vi "CSM - Module VI Reference.vi"(6 "Response Timeout (-2 Using Global Settings)":i32=-2, 7 "Current Module (\"\" to Generate an ID)":string, 8 "error in (no error)":errorcluster, 9 "Force? (F)":bool, 11 "CSM Name":string) -> (0 "error out":errorcluster, 3 "CSM Module VIRef":refnum<vi>)   [LabVIEW 2017, in "Communicable State Machine.lvlib"]
doc: "Obtains the VI Reference of the input module.\n\nThe following is the logic of this VI:\n- This VI queries and retrieves the CSM module's VI reference by sending a `VI Reference` synchronous message, so it has input parameters similar to the VI that sends synchronous messages.\n- This VI caches the VI reference of the CSM module queried during the current main program run in the background. When the same module is queried again and the retrieved VI reference is still valid, the cached VI reference is returned directly instead of sending another synchronous message query.\n- If you need to force a re-query of the module's VI reference, you can set <b>Force? (F)</b> to TRUE.\n\nBehavior for CSM in special operation modes:\n- <b>Worker Mode</b>: Returns the VI reference of the worker node handling the `VI Reference` message.\n- <b>Chain of Responsibility Mode</b>: Returns the VI reference of the first node of the CSM module in Chain of Responsibility Mode.\n- <b>System-Level Module</b>: Same as normal mode CSM. Returns the VI reference of the system-level module.\n\n\n> [!WARNING] <b>Multiple CSMs in a Single VI</b>\n>\n> - It is not recommended to place multiple (>=2) CSMs in a flat layout within a single VI. While this will not cause logical issues in the program, it will prevent the CSM Debug Console from loading all the inner and outer interfaces of the flat CSMs in that VI - only one will be loaded.\n\n\n-- <b>Controls</b> --\n- <b>Current Module (\"\" to Generate an ID)</b>: Tag for the querying CSM module. If empty, a unique ID is generated.\n- <b>CSM Name</b>: CSM module name.\n- <b>Force? (F)</b>: Whether to force a re-query of the module's VI reference. The default is FALSE.\n- <b>Response Timeout (-2 Using Global Settings)</b>: Timeout for synchronous calls. The default is -2, which uses the global setting. You can set the global timeout using the CSM - Set TMO of Sync-Reply VI.\n\n-- <b>Indicators</b> --\n- <b>CSM Module VIRef</b>: VI reference of the CSM module."
uses:
  Communicable State Machine.lvlib
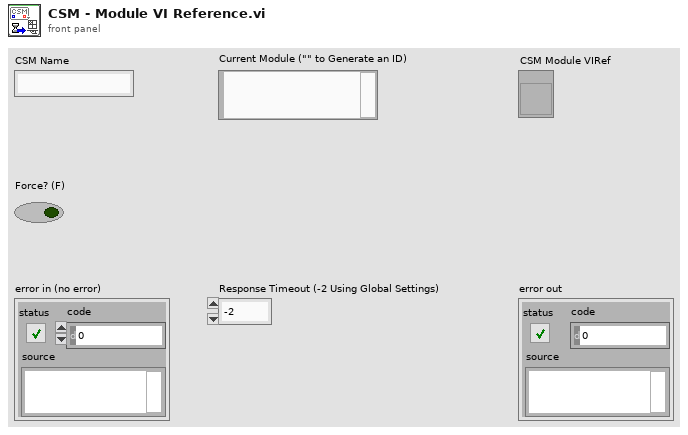
[diagram p1: front panel]
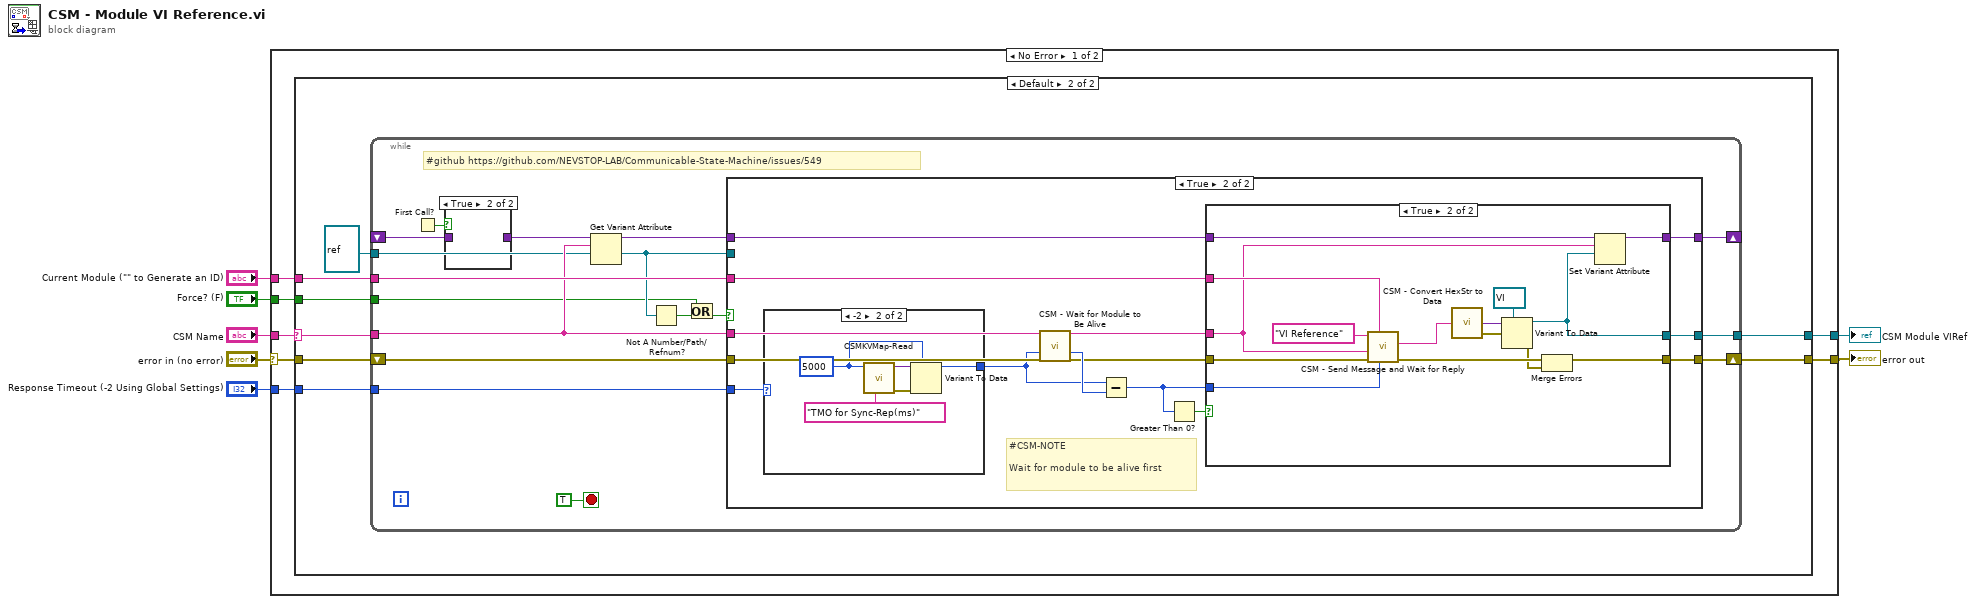
[diagram p0: block diagram]
diagram:
  n1 = case shown="No Error" "error in (no error)" {
    selector: "error in (no error)" -> [w12 w82]
    tunnel: "Response Timeout (-2 Using Global Settings)" -> [w14 _]
    tunnel: "Current Module (\"\" to Generate an ID)" -> [w13 _]
    tunnel: "CSM Name" -> [w11 _]
    tunnel: [w10 w82] -> w2
    tunnel: [w9 _] -> w3
    tunnel: "Force? (F)" -> [w8 _]
    frame No Error {
      n2 = case shown="Default" w11 {
        selector: w11 -> [_ w18]
        tunnel: w14 -> [_ w16]
        tunnel: w13 -> [_ w23]
        tunnel: w12 -> [w15 w17]
        tunnel: [w15 w22] -> w10
        tunnel: [_ w21] -> w9
        tunnel: w8 -> [_ w19]
        frame "" {
        }
        frame Default {
          n3 = while {
            tunnel: w16 -> [w40]
            tunnel: w23 -> [w39]
            tunnel: w18 -> [w34]
            tunnel: [w36] -> w21
            shift-right: [w37] -> w22
            shift-left: w17 -> [w38]
            shift-right: [w31] -> _
            shift-left: _ -> [w24]
            tunnel: refnum<vi> refnum ("CSM Module VIRef") -> [w33]
            tunnel: w19 -> [w27]
            stop <- TRUE stop-if-true
            # "#github https://github.com/NEVSTOP-LAB/Communicable-State-Machine/issues/549"
            n4 = First Call?() -> (First Call?: T/F=w26:bool)
            n5 = case shown="True" w26 {
              tunnel: [w41 _] -> w25
              tunnel: w24 -> [w41 _]
              frame False {
              }
              frame True {
              }
            }
            n6 = Get Variant Attribute(Variant=w25, name=w34, default value (empty Variant)=w33) -> (duplicate Variant=w30:variant, value=w29:refnum<vi>)  [unwired: 1 in, 2 out]
            n7 = Not A Number/Path/Refnum?(number/path/refnum=w29) -> (NaN/Path/Refnum?=w32:bool)
            n8 = Or(x=w27, y=w32) -> (x .or. y?=w28:bool)
            n9 = case shown="True" w28 {
              tunnel: w40 -> [_ w46]
              tunnel: w39 -> [_ w58]
              tunnel: w38 -> [w42 w52]
              tunnel: [w42 w57] -> w37
              tunnel: [w43 w54] -> w36
              tunnel: w34 -> [_ w50]
              tunnel: [w44 w55] -> w31
              tunnel: w30 -> [w44 w56]
              tunnel: w29 -> [w43 _]
              frame False {
              }
              frame True {
                # "#CSM-NOTE\n\nWait for module to be alive first"
                n10 = case shown="-2" w46 {
                  selector: w46 -> [w59 _]
                  tunnel: [w59 w60] -> w45
                  frame 0, Default {
                  }
                  frame -2 {
                    w61 = 5000 ("max queue size (-1, unlimited)")
                    n11 = call "CSMKVMap-Read.vi"("name"="TMO for Sync-Rep(ms)", "default value (empty variant)"=w61) -> ("Error out"=w64:errorcluster, "value"=w63:variant)  [unwired: 6 in]
                    n12 = Variant To Data(error in=w64, type=w61, Variant=w63) -> (data=w60:i32)  [unwired: 1 out]
                  }
                }
                n13 = call "CSM - Wait for Module to Be Alive.vi"("CSM Name"=w50, "Wait (5000 ms)"=w45, "error in (no error)"=w52) -> ("CSM Name (Dup)"=w49:string, "Waited (ms)"=w53:u32, "error out"=w51:errorcluster)  [unwired: 10 in]
                n14 = Subtract(x=w45, y=w53) -> (x-y=w48:u32)
                n15 = Greater Than 0?(x=w48) -> (x > 0?=w47:bool)
                n16 = case shown="True" w47 {
                  tunnel: w58 -> [_ w81]
                  tunnel: [w65 w80] -> w57
                  tunnel: w56 -> [w66 w79]
                  tunnel: [w66 w78] -> w55
                  tunnel: [_ w77] -> w54
                  tunnel: w51 -> [w65 w69]
                  tunnel: w49 -> [_ w68]
                  tunnel: w48 -> [_ w67]
                  frame False {
                  }
                  frame True {
                    n17 = call "CSM - Send Message and Wait for Reply.vi"("Response Timeout (-2 Using Global Settings)"=w67, "Current Module (\"\" to Generate an ID)"=w81, "Error In (No Error)"=w69, "Target Module"=w68, "State"="VI Reference") -> ("error out"=w75:errorcluster, "Response"=w74:string)  [unwired: 4 in, 1 out]
                    n18 = call "CSM - Convert HexStr to Data.vi"("HEX String"=w74) -> ("Variant"=w72:variant, "error out"=w73:errorcluster)  [unwired: 7 in]
                    n19 = Variant To Data(error in=w73, type=refnum<vi> refnum ("Current VI Reference"), Variant=w72) -> (data=w77:refnum<vi>, error out=w70:errorcluster)
                    n20 = Merge Errors(w75, w70) -> (w80:errorcluster)
                    n21 = Set Variant Attribute(Variant=w79, name=w68, value=w77) -> (Variant out=w78:variant)  [unwired: 1 in, 2 out]
                  }
                }
              }
            }
          }
        }
      }
    }
    frame Error {
    }
  }
  "error out" <- w2
  "CSM Module VIRef" <- w3
